vi "GetVoltageInfo.vi"() -> (1 "VoltageInfo":string[](array[string]), 2 "Error":bool)   [LabVIEW 2014]
panel:
  out "ClockPins":string[](array[string])
  out "VideoPins":string[](array[string])
  out "ClockInfo":string[](array[string])
  out "VideoInfo":string[](array[string])
  out "ClockMaximums":string[](array[string])
  out "ClockMinimums":string[](array[string])
  out "ClockVoltages":string[](array[string])
  out "ClockNames":string[](array[string])
  out "VideoMaximums":string[](array[string])
  out "VideoMinimums":string[](array[string])
  out "VideoVoltages":string[](array[string])
  out "VideoNames":string[](array[string])
  out "VideoBoards":string[](array[string])
  out "ClockBoards":string[](array[string])
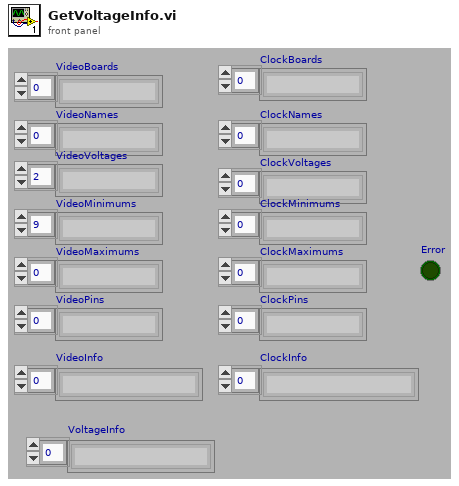
[diagram p1: front panel]
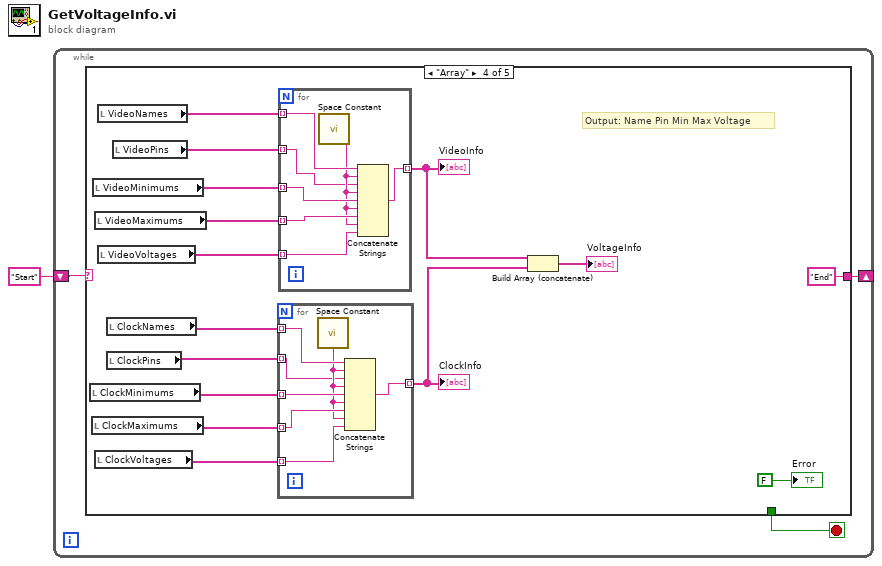
[diagram p0: block diagram]
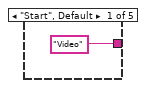
[diagram p2: hidden frame]
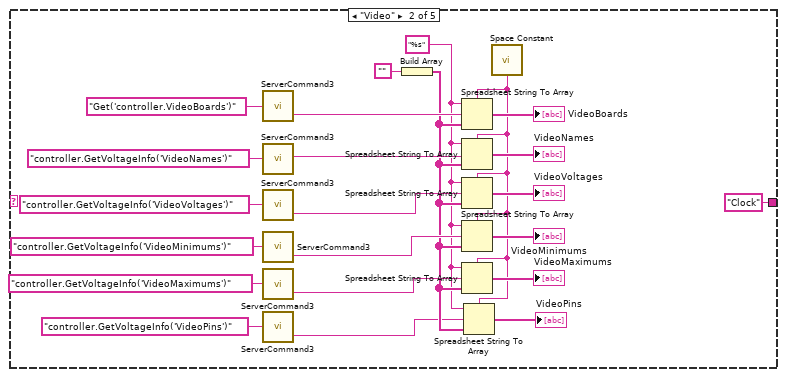
[diagram p3: hidden frame]
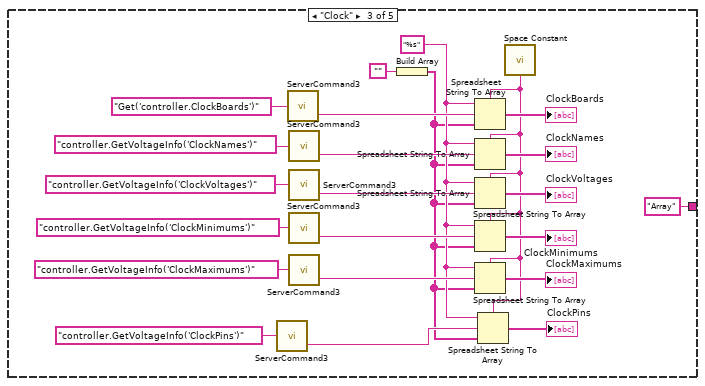
[diagram p4: hidden frame]
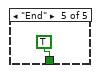
[diagram p5: hidden frame]
diagram:
  n1 = while {
    shift-right: [w4] -> _
    shift-left: "Start" ("Command") -> [w3]
    stop <- w2 stop-if-true
    n2 = case shown="\"Array\"" w3 {
      tunnel: ["Video" ("Command") "Clock" ("Command") "Array" ("Command") "End" ("Command") _] -> w4
      tunnel: [_ _ _ _ TRUE] -> w2
      frame "Start", Default {
      }
      frame "Video" {
        w7 = "%s" ("format string")
        n3 = call "ServerCommand3.vi"("Command"="Get('controller.VideoBoards')") -> ("Reply"=w21:string)  [unwired: 1 out]
        n4 = call "ServerCommand3.vi"("Command"="controller.GetVoltageInfo('VideoNames')") -> ("Reply"=w15:string)  [unwired: 1 out]
        n5 = call "ServerCommand3.vi"("Command"="controller.GetVoltageInfo('VideoVoltages')") -> ("Reply"=w14:string)  [unwired: 1 out]
        n6 = call "ServerCommand3.vi"("Command"="controller.GetVoltageInfo('VideoMinimums')") -> ("Reply"=w13:string)  [unwired: 1 out]
        n7 = call "ServerCommand3.vi"("Command"="controller.GetVoltageInfo('VideoMaximums')") -> ("Reply"=w12:string)  [unwired: 1 out]
        n8 = call "ServerCommand3.vi"("Command"="controller.GetVoltageInfo('VideoPins')") -> ("Reply"=w8:string)  [unwired: 1 out]
        n9 = Build Array("") -> (w10:string[])
        n10 = call <vilib>:"Space Constant.vi"() -> ("String"=w6:string)
        n11 = Spreadsheet String To Array(delimiter (Tab)=w6, format string=w7, spreadsheet string=w21, array type (2D Dbl)=w10) -> (array=→"VideoBoards":string[])
        n12 = Spreadsheet String To Array(delimiter (Tab)=w6, format string=w7, spreadsheet string=w15, array type (2D Dbl)=w10) -> (array=→"VideoNames":string[])
        n13 = Spreadsheet String To Array(delimiter (Tab)=w6, format string=w7, spreadsheet string=w14, array type (2D Dbl)=w10) -> (array=→"VideoVoltages":string[])
        n14 = Spreadsheet String To Array(delimiter (Tab)=w6, format string=w7, spreadsheet string=w13, array type (2D Dbl)=w10) -> (array=→"VideoMinimums":string[])
        n15 = Spreadsheet String To Array(delimiter (Tab)=w6, format string=w7, spreadsheet string=w12, array type (2D Dbl)=w10) -> (array=→"VideoMaximums":string[])
        n16 = Spreadsheet String To Array(delimiter (Tab)=w6, format string=w7, spreadsheet string=w8, array type (2D Dbl)=w10) -> (array=→"VideoPins":string[])
      }
      frame "Clock" {
        w32 = "%s" ("format string")
        n17 = call "ServerCommand3.vi"("Command"="controller.GetVoltageInfo('ClockPins')") -> ("Reply"=w33:string)  [unwired: 1 out]
        n18 = call "ServerCommand3.vi"("Command"="Get('controller.ClockBoards')") -> ("Reply"=w44:string)  [unwired: 1 out]
        n19 = call "ServerCommand3.vi"("Command"="controller.GetVoltageInfo('ClockNames')") -> ("Reply"=w43:string)  [unwired: 1 out]
        n20 = call "ServerCommand3.vi"("Command"="controller.GetVoltageInfo('ClockVoltages')") -> ("Reply"=w42:string)  [unwired: 1 out]
        n21 = call "ServerCommand3.vi"("Command"="controller.GetVoltageInfo('ClockMinimums')") -> ("Reply"=w41:string)  [unwired: 1 out]
        n22 = call "ServerCommand3.vi"("Command"="controller.GetVoltageInfo('ClockMaximums')") -> ("Reply"=w40:string)  [unwired: 1 out]
        n23 = Build Array("") -> (w31:string[])
        n24 = call <vilib>:"Space Constant.vi"() -> ("String"=w29:string)
        n25 = Spreadsheet String To Array(delimiter (Tab)=w29, format string=w32, spreadsheet string=w44, array type (2D Dbl)=w31) -> (array=→"ClockBoards":string[])
        n26 = Spreadsheet String To Array(delimiter (Tab)=w29, format string=w32, spreadsheet string=w43, array type (2D Dbl)=w31) -> (array=→"ClockNames":string[])
        n27 = Spreadsheet String To Array(delimiter (Tab)=w29, format string=w32, spreadsheet string=w42, array type (2D Dbl)=w31) -> (array=→"ClockVoltages":string[])
        n28 = Spreadsheet String To Array(delimiter (Tab)=w29, format string=w32, spreadsheet string=w41, array type (2D Dbl)=w31) -> (array=→"ClockMinimums":string[])
        n29 = Spreadsheet String To Array(delimiter (Tab)=w29, format string=w32, spreadsheet string=w40, array type (2D Dbl)=w31) -> (array=→"ClockMaximums":string[])
        n30 = Spreadsheet String To Array(delimiter (Tab)=w29, format string=w32, spreadsheet string=w33, array type (2D Dbl)=w31) -> (array=→"ClockPins":string[])
      }
      frame "Array" {
        # "Output: Name Pin Min Max Voltage"
        n31 = local read "ClockMinimums"() -> (w60:string[])
        n32 = local read "ClockMaximums"() -> (w59:string[])
        n33 = local read "VideoMinimums"() -> (w64:string[])
        n34 = local read "VideoMaximums"() -> (w63:string[])
        n35 = local read "ClockVoltages"() -> (w58:string[])
        n36 = local read "VideoNames"() -> (w65:string[])
        n37 = local read "VideoVoltages"() -> (w62:string[])
        n38 = local read "ClockNames"() -> (w61:string[])
        n39 = local read "ClockPins"() -> (w56:string[])
        n40 = local read "VideoPins"() -> (w55:string[])
        n41 = for {
          tunnel: w61 -> [w69] mode=indexing
          tunnel: w60 -> [w73] mode=indexing
          tunnel: w59 -> [w72] mode=indexing
          tunnel: w58 -> [w71] mode=indexing
          tunnel: [w70] -> w53 mode=indexing
          tunnel: w56 -> [w67] mode=indexing
          n42 = call <vilib>:"Space Constant.vi"() -> ("String"=w68:string)
          n43 = Concatenate Strings(w69, w68, w67, w68, w73, w68, w72, w68, w71) -> (w70:string)
        }
        "ClockInfo" <- w53
        n44 = for {
          tunnel: w65 -> [w76] mode=indexing
          tunnel: w64 -> [w80] mode=indexing
          tunnel: w63 -> [w79] mode=indexing
          tunnel: w62 -> [w78] mode=indexing
          tunnel: [w77] -> w54 mode=indexing
          tunnel: w55 -> [w74] mode=indexing
          n45 = call <vilib>:"Space Constant.vi"() -> ("String"=w75:string)
          n46 = Concatenate Strings(w76, w75, w74, w75, w80, w75, w79, w75, w78) -> (w77:string)
        }
        "VideoInfo" <- w54
        n47 = Build Array (concatenate)(w54, w53) -> (→"VoltageInfo":string[])
        "Error" <- FALSE ("Error")
      }
      frame "End" {
      }
    }
  }
